vi "[del]Open Dialog.vi"(8 "error in (no error)":errorcluster caption="错误输入（无错误）") -> (0 "error out":errorcluster caption="错误输出", 3 "Open?":bool)   [LabVIEW 2011]
uses:
  CAN FD.lvlib
panel:
  in  "Tab":enum32{"CAN0", "CAN1"}(tab)
  in  "Ch0":T1={"Enable"=TRUE, "Terminal"=0, "Param"={"abitbaud"=500000, "dbitbaud"=500000, "CustomBaud"=FALSE, "CustomBd"="", "Mode"=0}} {"Param"."dbitbaud" items=["5Mbps"=5000000, "4Mbps"=4000000, "2Mbps"=2000000, "1Mbps"=1000000, "800kbps"=800000, "500kbps"=500000, "250kbps"=250000, "125kbps"=125000, "100kbps"=100000]; "Param"."abitbaud" items=["1Mbps"=1000000, "800kbps"=800000, "500kbps"=500000, "250kbps"=250000, "125kbps"=125000, "100kbps"=100000, "50kbps"=50000]; "Param"."Mode" items=["正常", "只听"]; "Terminal" items=["禁用", "启用"]}
  in  "Ch1":T1={"Enable"=TRUE, "Terminal"=0, "Param"={"abitbaud"=500000, "dbitbaud"=500000, "CustomBaud"=FALSE, "CustomBd"="", "Mode"=0}} {"Param"."dbitbaud" items=["5Mbps"=5000000, "4Mbps"=4000000, "2Mbps"=2000000, "1Mbps"=1000000, "800kbps"=800000, "500kbps"=500000, "250kbps"=250000, "125kbps"=125000, "100kbps"=100000]; "Param"."abitbaud" items=["1Mbps"=1000000, "800kbps"=800000, "500kbps"=500000, "250kbps"=250000, "125kbps"=125000, "100kbps"=100000, "50kbps"=50000]; "Param"."Mode" items=["正常", "只听"]; "Terminal" items=["禁用", "启用"]}
  in  "Cancel":bool
  in  "OK":bool
  in  "Index":u32(ring) caption="索引" items=["0", "1", "2", "3", "4", "5", "6", "7", "8"]
  in  "Type":u32(ring)=41 caption="CAN卡型号" items=["USBCANFD-200U"=41, "USBCANFD-100U"=42]
  # "通道参数"
  # "通道参数"
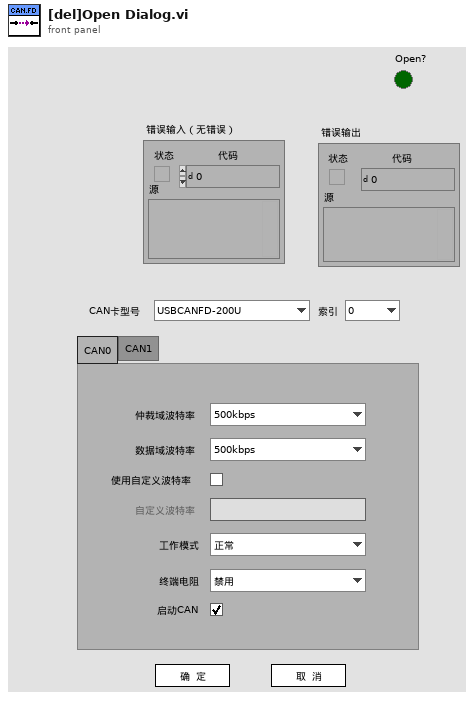
[diagram p1: front panel]
types:
  T1 = cluster{"Enable":bool, "Terminal":u32, "Param":cluster{"abitbaud":u32, "dbitbaud":u32, "CustomBaud":bool, "CustomBd":string, "Mode":u8}}
  T2 = cluster{"Enable":bool, "Terminal":u32, "Param":cluster{"abitbaud":u32, "dbitbaud":u32, "CustomBaud":bool, "CustomBd":string, "Mode":u8}}[]
  T3 = cluster{"abitbaud":u32, "dbitbaud":u32, "CustomBaud":bool, "CustomBd":string, "Mode":u8}
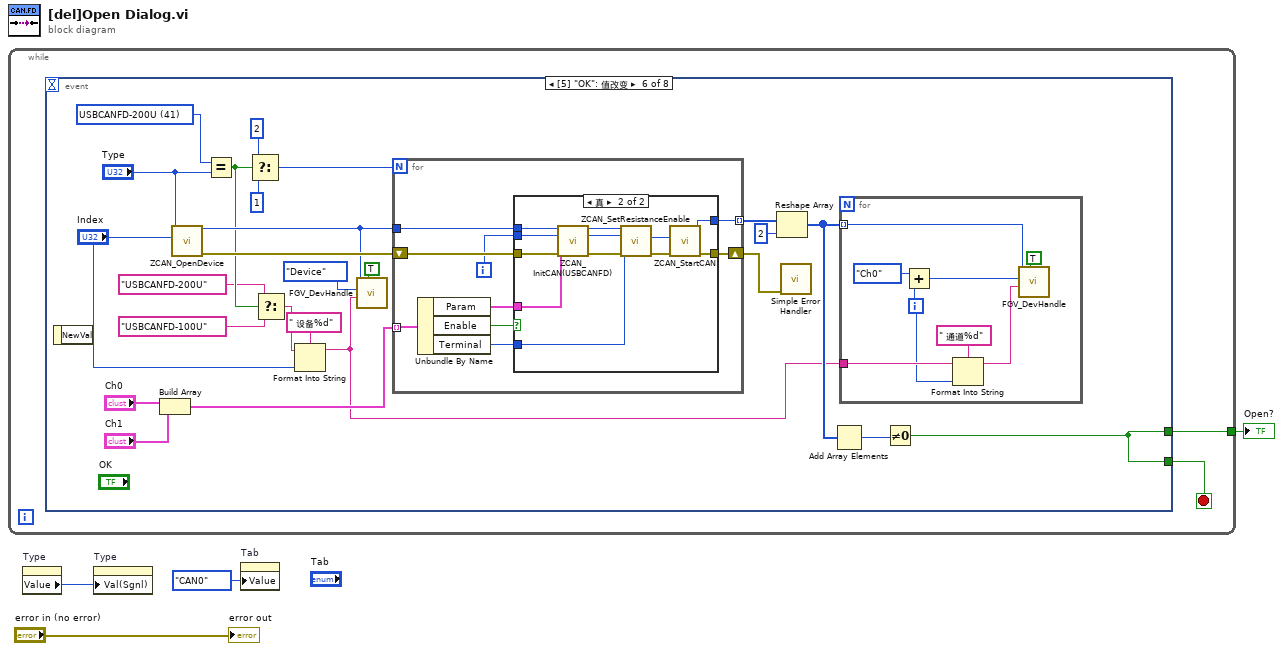
[diagram p0: block diagram]
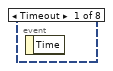
[diagram p2: hidden frame]
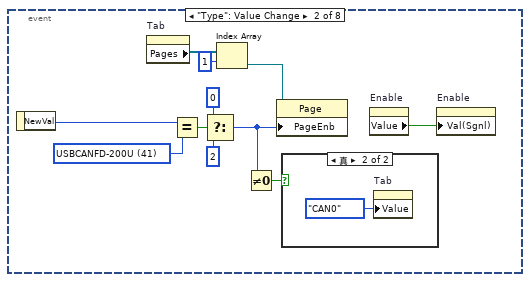
[diagram p3: hidden frame]
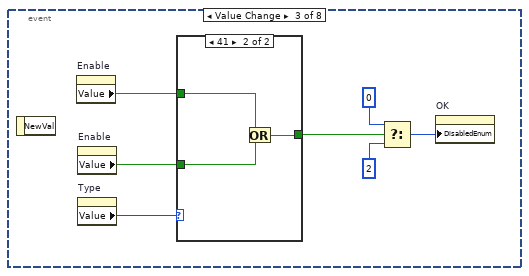
[diagram p5: hidden frame]
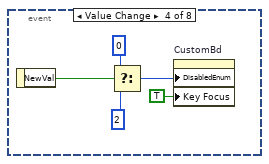
[diagram p7: hidden frame]
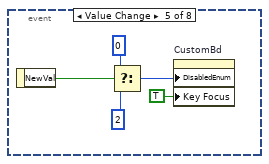
[diagram p8: hidden frame]
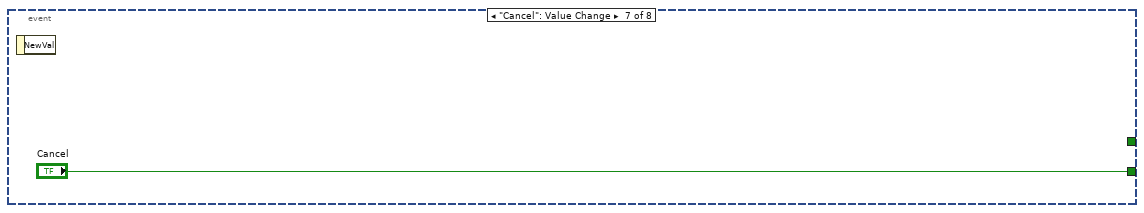
[diagram p10: hidden frame]
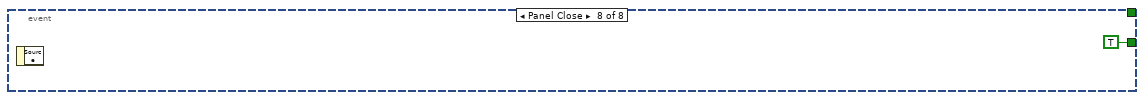
[diagram p11: hidden frame]
diagram:
  n1 = while {
    tunnel: [w5] -> w2
    stop <- w6 stop-if-true
    n2 = event shown="[5] \"OK\": 值改变" {
      selector: _ -> [_ _ _ _ _ _ _ _]
      dyn-events: _ -> [_ _ _ _ _ _ _ _]
      timeout: _ -> [_ _ _ _ _ _ _ _]
      tunnel: [_ _ _ _ _ w47 "Cancel" TRUE ("Cancel")] -> w6
      tunnel: [_ _ _ _ _ w47 _ _] -> w5
      event Timeout {
        n3 = event-data() -> ()  [unwired: 1 in, 1 out]
      }
      event "Type": Value Change {
        w16 = u32 41 items=["USBCANFD-200U"=41, "USBCANFD-100U"=42] ("Type")
        n4 = event-data() -> ("NewVal"=w17:u32)  [unwired: 1 in]
        n5 = property on="Tab" class="TabCtl (严格)"() -> ("Pages"=w12:refnum<vi>[])  [unwired: 2 in, 2 out]
        n6 = Equal?(x=w17, y=w16) -> (x = y?=w15:bool)
        n7 = Select(t=0, s=w15, f=2) -> (s? t:f=w9:i32)
        n8 = Index Array(array=w12, index=1 ("索引")) -> (element=w10:refnum<vi>)
        n9 = Not Equal To 0?(x=w9) -> (x != 0?=w8:bool)
        n10 = property class="Page"(reference=w10, "PageEnb"=w9) -> ()  [unwired: 1 in, 2 out]
        n11 = case shown="真" w8 {
          frame False {
          }
          frame True {
            n12 = property on="Tab" class="TabCtl (严格)"("Value"=enum32{"CAN0", "CAN1"}."CAN0" ("Tab")) -> ()  [unwired: 2 in, 2 out]
          }
        }
        n13 = property on="Enable" class="Bool (严格)"() -> ("Value"=w7:bool)  [unwired: 2 in, 2 out]
        n14 = property on="Enable" class="Bool (严格)"("Val(Sgnl)"=w7) -> ()  [unwired: 2 in, 2 out]
      }
      event "Ch1.Enable", "Ch0.Enable": Value Change {
        n15 = event-data() -> ()  [unwired: 1 in, 1 out]
        n16 = property on="Enable" class="Bool (严格)"() -> ("Value"=w20:bool)  [unwired: 2 in, 2 out]
        n17 = property on="Enable" class="Bool (严格)"() -> ("Value"=w19:bool)  [unwired: 2 in, 2 out]
        n18 = property on="Type" class="Ring (严格)"() -> ("Value"=w25:u32)  [unwired: 2 in, 2 out]
        n19 = case shown="41" w25 {
          tunnel: [w26 w29] -> w21
          tunnel: w20 -> [w26 w28]
          tunnel: w19 -> [_ w27]
          frame 42, Default {
          }
          frame 41 {
            n20 = Or(x=w28, y=w27) -> (x .or. y?=w29:bool)
          }
        }
        n21 = Select(t=0, s=w21, f=2) -> (s? t:f=w22:i32)
        n22 = property on="OK" class="Bool"("DisabledEnum"=w22) -> ()  [unwired: 2 in, 2 out]
      }
      event "Ch0.Param.CustomBaud": Value Change {
        n23 = event-data() -> ("NewVal"=w34:bool)  [unwired: 1 in]
        n24 = Select(t=0, s=w34, f=2) -> (s? t:f=w31:i32)
        n25 = property on="CustomBd" class="Str"("DisabledEnum"=w31, "Key Focus"=TRUE ("键选中")) -> ()  [unwired: 2 in, 2 out]
      }
      event "Ch1.Param.CustomBaud": Value Change {
        n26 = event-data() -> ("NewVal"=w39:bool)  [unwired: 1 in]
        n27 = Select(t=0, s=w39, f=2) -> (s? t:f=w36:i32)
        n28 = property on="CustomBd" class="Str"("DisabledEnum"=w36, "Key Focus"=TRUE ("键选中")) -> ()  [unwired: 2 in, 2 out]
      }
      event "OK": Value Change {
        w60 = u32 41 items=["USBCANFD-200U"=41, "USBCANFD-100U"=42] ("Type")
        n29 = event-data() -> ()  [unwired: 1 in, 1 out]
        n30 = Build Array("Ch0", "Ch1") -> (w61:T2)
        n31 = call "ZCAN_OpenDevice.vi"("device_index"="Index", "device_type"="Type") -> ("error out"=w64:errorcluster, "DEVICE_HANDLE"=w55:u32)  [unwired: 8 in]
        n32 = Equal?(x=w60, y="Type") -> (x = y?=w46:bool)
        n33 = Select(t=2, s=w46, f=1) -> (s? t:f=w58:i32)
        n34 = Select(t="USBCANFD-200U", s=w46, f="USBCANFD-100U") -> (s? t:f=w43:string)
        n35 = Format Into String(format string=" 设备%d" ("格式字符串"), initial string=w43, "Index") -> (resulting string=w40:string)  [unwired: 1 in, 1 out]
        n36 = call "FGV_DevHandle.vi"("Set"=TRUE, "Name"=w40, "Type"=enum16{"Device", "Ch0", "Ch1"}."Device", "handle"=w55) -> ()  [unwired: 5 in, 3 out]
        n37 = for {
          N: w58 -> [_]
          tunnel: w55 -> [w80]
          tunnel: w61 -> [w78] mode=indexing
          shift-right: [w79] -> w48
          shift-left: w64 -> [w81]
          tunnel: [w73] -> w52 mode=indexing
          i -> [w74]
          n38 = Unbundle By Name(w78) -> ("Param"=w77:T3, "Enable"=w76:bool, "Terminal"=w75:u32)
          n39 = case shown="真" w76 {
            tunnel: w81 -> [w82 w89]
            tunnel: w80 -> [_ w88]
            tunnel: [w82 w87] -> w79
            tunnel: w77 -> [_ w86]
            tunnel: w75 -> [_ w85]
            tunnel: w74 -> [_ w84]
            tunnel: [_ w83] -> w73
            frame False {
            }
            frame True {
              n40 = call "ZCAN_InitCAN(USBCANFD).vi"("device_hande"=w88, "can_index"=w84, "ZCAN_InitCAN_Setting_USBCANFD"=w86, "error in (no error)"=w89) -> ("can_index_handle"=w91:u32, "error out"=w93:errorcluster)  [unwired: 10 in]
              n41 = call "ZCAN_SetResistanceEnable.vi"("error in (no error)"=w93, "enable"=w85, "can_index"=w84, "can_index_handle"=w91) -> ("error out"=w92:errorcluster, "can_index_handle(out)"=w90:u32)  [unwired: 6 in]
              n42 = call "ZCAN_StartCAN.vi"("error in (no error)"=w92, "can_index_handle"=w90) -> ("error out"=w87:errorcluster, "can_index_handle(out)"=w83:u32)  [unwired: 7 in, 1 out]
            }
          }
        }
        n43 = Reshape Array(w52, 2 ("维数大小")) -> (w50:u32[])
        n44 = call <vilib>:"Simple Error Handler.vi"("error in (no error)"=w48) -> ()  [unwired: 4 in, 5 out]
        n45 = Add Array Elements(numeric array=w50) -> (sum=w49:u32)
        n46 = for {
          tunnel: w50 -> [w71] mode=indexing
          tunnel: w40 -> [w68]
          i -> [w65]
          n47 = Add(x=enum16{"Device", "Ch0", "Ch1"}."Ch0" ("Type"), y=w65) -> (x+y=w70:i32)
          n48 = Format Into String(format string=" 通道%d" ("格式字符串"), initial string=w68, w65) -> (resulting string=w66:string)  [unwired: 1 in, 1 out]
          n49 = call "FGV_DevHandle.vi"("Set"=TRUE, "Name"=w66, "Type"=w70, "handle"=w71) -> ()  [unwired: 5 in, 3 out]
        }
        n50 = Not Equal To 0?(x=w49) -> (x != 0?=w47:bool)
      }
      event "Cancel": Value Change {
        n51 = event-data() -> ()  [unwired: 1 in, 1 out]
      }
      event Panel Close {
        n52 = event-data() -> ()  [unwired: 1 in, 1 out]
      }
    }
  }
  "Open?" <- w2
  n53 = property on="Type" class="Ring (严格)"() -> ("Value"=w3:u32)  [unwired: 2 in, 2 out]
  n54 = property on="Type" class="Ring (严格)"("Val(Sgnl)"=w3) -> ()  [unwired: 2 in, 2 out]
  n55 = property on="Tab" class="TabCtl (严格)"("Value"=enum32{"CAN0", "CAN1"}."CAN0" ("Tab")) -> ()  [unwired: 2 in, 2 out]
  "error out" <- "error in (no error)"
